vi "Get NEC Call Chain.vi"(8 "error in (no error)":errorcluster) -> (0 "error out":errorcluster, 5 "Call Chain":string[](array[string]))   [LabVIEW 2016, in "Stream Error.lvlib" / "Error Interface.lvclass"]
doc: "--\nCopyright © 2017 Composed SystemsI All rights reserved.\n\nAuthor: Jon McBee <jon.mcbee@composed.io>\n\nThis library is provided \"AS IS\" ,WITHOUT WARRANTIES OR\nCONDITIONS OF ANY KIND, either express or implied.\n\nComposed Systems -- composed.io\n\nStream 0.0.1.1\nJon McBee - Composed Systems\nCopyright (c) 2017, Composed Systems"
uses:
  <userlib>/Composed Systems/Stream/Error/Classes/Error Interface/Error Interface.lvclass
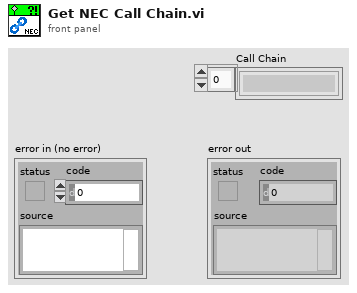
[diagram p1: front panel]
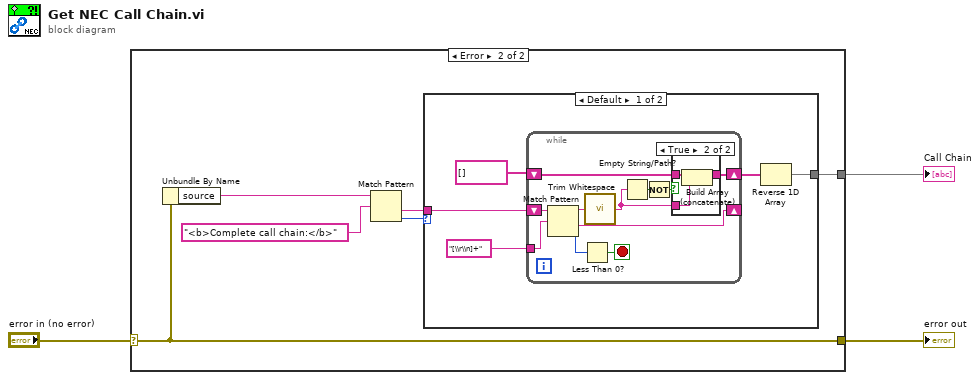
[diagram p0: block diagram]
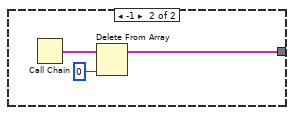
[diagram p4: hidden frame]
diagram:
  n1 = case shown="Error" "error in (no error)" {
    selector: "error in (no error)" -> [w4 w10]
    tunnel: [w4 w10] -> w2
    tunnel: [_ w5] -> w1
    frame No Error {
    }
    frame Error {
      n2 = Unbundle By Name(w10) -> ("source"=w8:string)
      n3 = Match Pattern(string=w8, regular expression="<b>Complete call chain:</b>") -> (after substring=w6:string, offset past match=w7:i32)  [unwired: 1 in, 2 out]
      n4 = case shown="Default" w7 {
        tunnel: w6 -> [w13 _]
        tunnel: [w11 w31] -> w5
        frame Default {
          n5 = while {
            shift-right: [w25] -> _
            shift-left: w13 -> [w26]
            tunnel: "[\\r\\n]+" ("regular expression") -> [w18]
            shift-right: [w16] -> w14
            shift-left: string[] [] ("Array") -> [w17]
            stop <- w23 stop-if-true
            n6 = Match Pattern(string=w26, regular expression=w18) -> (before substring=w22:string, after substring=w25:string, offset past match=w24:i32)  [unwired: 1 in, 1 out]
            n7 = Less Than 0?(x=w24) -> (x < 0?=w23:bool)
            n8 = call <vilib>:"Trim Whitespace.vi"("string"=w22) -> ("trimmed string"=w20:string)  [unwired: 1 in]
            n9 = Empty String/Path?(string/path=w20) -> (empty?=w19:bool)
            n10 = Not(x=w19) -> (.not. x?=w21:bool)
            n11 = case shown="True" w21 {
              tunnel: w17 -> [w27 w29]
              tunnel: w20 -> [_ w28]
              tunnel: [w27 w30] -> w16
              frame False {
              }
              frame True {
                n12 = Build Array (concatenate)(w29, w28) -> (w30:string[])
              }
            }
          }
          n13 = Reverse 1D Array(array=w14) -> (reversed array=w11:string[])
        }
        frame -1 {
          n14 = Call Chain() -> (call chain=w33:string[])
          n15 = Delete From Array(array=w33, index=0) -> (array with subset deleted=w31:string[])  [unwired: 1 in, 1 out]
        }
      }
    }
  }
  "error out" <- w2
  "Call Chain" <- w1
